vi "Update Status Table by Reference.vi"(8 "error in (no error)":errorcluster, 10 "Plugin Info Array":T1[](array[typedef]) {"Node Status"."Monitor Doubles"."4" format="%#_9g"; "Node Status"."Monitor Doubles"."3" format="%#_9g"; "Node Status"."Monitor Doubles"."2" format="%#_9g"; "Node Status"."Monitor Doubles"."1" format="%#_9g"; "Node Status"."Timing Statistics (us)"."Period"."Avg" format="%_6g"}, 11 "Table Control in":refnum<vi>) -> (0 "error out":errorcluster)   [LabVIEW 2021, in "CIF_UI.lvclass"]
uses:
  CIF_UI.lvclass
  CIFCore/Common/Typedef/PluginInfo.ctl
  CIFCore/Common/Typedef/Version Simple.ctl
  CIFCore/Common/Typedef/gRPC Reported Plugin Status.ctl
  CIFCore/Common/Typedef/Plugin State.ctl
  CIFCore/Common/Typedef/Timing Statistics.ctl
  CIFCore/Common/Typedef/Timing Stats Base.ctl
  CIFCore/Common/Typedef/FIFO Statistics.ctl
  CIFCore/Common/Typedef/Simple Error.ctl
  CIFCore/Common/Typedef/Monitor Doubles.ctl
  CIFCore/Common/Typedef/Monitor U64.ctl
  CIFCore/Common/Typedef/Monitor I64.ctl
  CIFCore/Common/CIFCoreCommon.lvlib
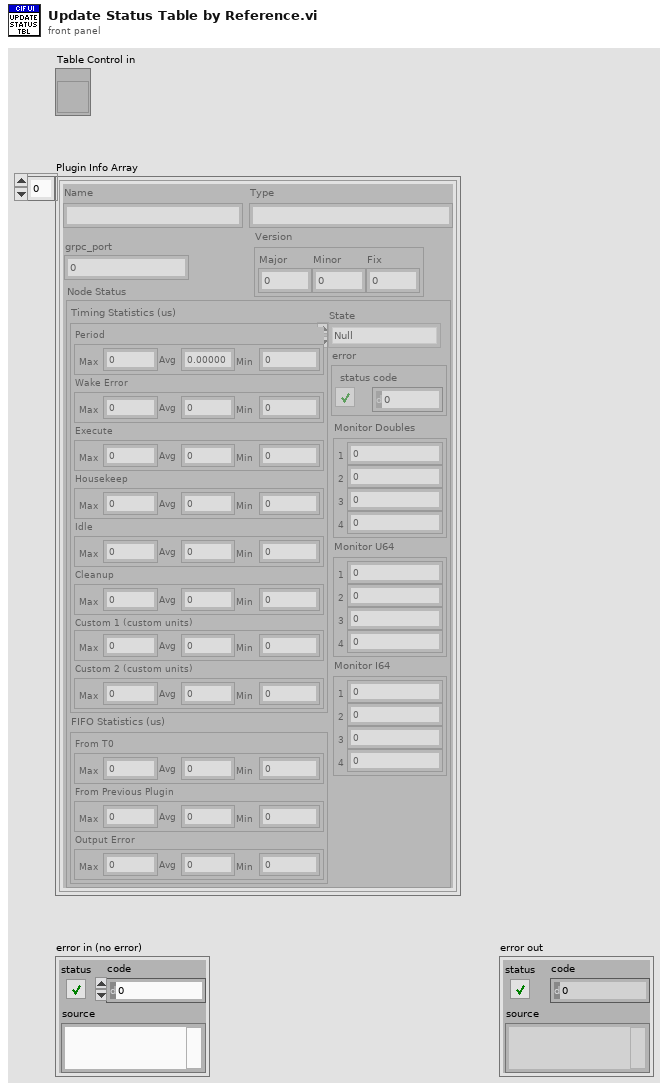
[diagram p1: front panel]
types:
  T1 = typedef "CIFCoreCommon.lvlib/PluginInfo.ctl" = cluster{"Name":string, "Type":string, "grpc_port":i32, "Version":T2, "Node Status":T3}
  T2 = typedef "CIFCoreCommon.lvlib/Version Simple.ctl" = cluster{"Major":i32, "Minor":i32, "Fix":i32}
  T3 = typedef "CIFCoreCommon.lvlib/gRPC Reported Plugin Status.ctl" = cluster{"State":T4, "Timing Statistics (us)":T5, "FIFO Statistics (us)":T7, "error":T8, "Monitor Doubles":T9, "Monitor U64":T10, "Monitor I64":T11}
  T4 = typedef "CIFCoreCommon.lvlib/Plugin State.ctl" = enum32{"Null", "Creating", "Listening", "Running", "CleaningUp", "Destroying"}
  T5 = typedef "CIFCoreCommon.lvlib/Timing Statistics.ctl" = cluster{"Period":T6, "Wake Error":T6, "Execute":T6, "Housekeep":T6, "Idle":T6, "Cleanup":T6, "Custom 1 (custom units)":T6, "Custom 2 (custom units)":T6}
  T6 = typedef "CIFCoreCommon.lvlib/Timing Stats Base.ctl" = cluster{"Max":i64, "Avg":dbl, "Min":i64}
  T7 = typedef "CIFCoreCommon.lvlib/FIFO Statistics.ctl" = cluster{"From T0":T6, "From Previous Plugin":T6, "Output Error":T6}
  T8 = typedef "CIFCoreCommon.lvlib/Simple Error.ctl" = cluster{"status":bool, "code":i32}
  T9 = typedef "CIFCoreCommon.lvlib/Monitor Doubles.ctl" = cluster{"1":dbl, "2":dbl, "3":dbl, "4":dbl}
  T10 = typedef "CIFCoreCommon.lvlib/Monitor U64.ctl" = cluster{"1":u64, "2":u64, "3":u64, "4":u64}
  T11 = typedef "CIFCoreCommon.lvlib/Monitor I64.ctl" = cluster{"1":i64, "2":i64, "3":i64, "4":i64}
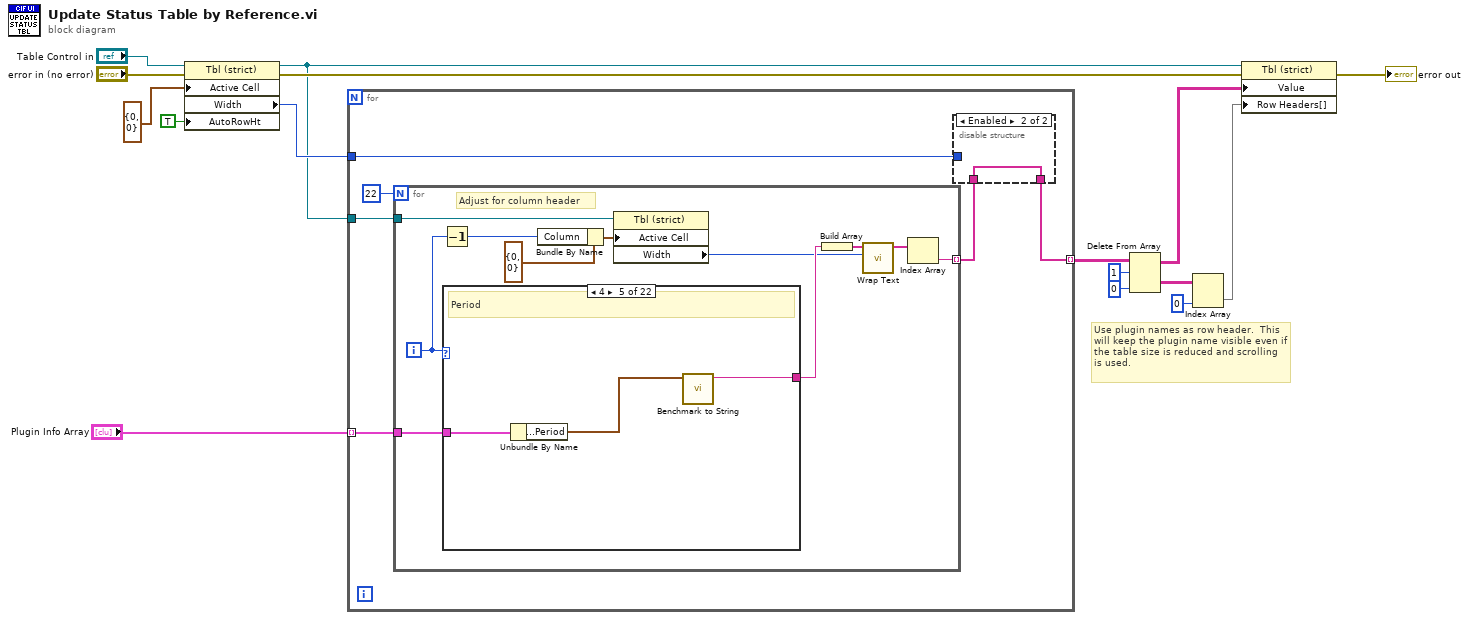
[diagram p0: block diagram]
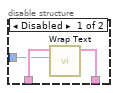
[diagram p2: hidden frame]
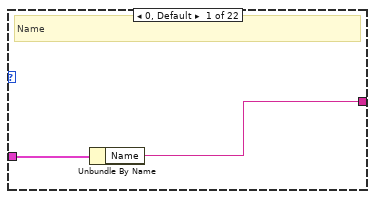
[diagram p3: hidden frame]
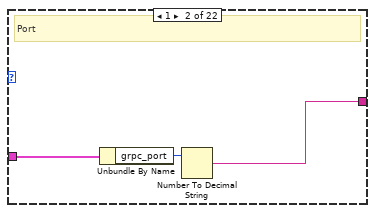
[diagram p4: hidden frame]
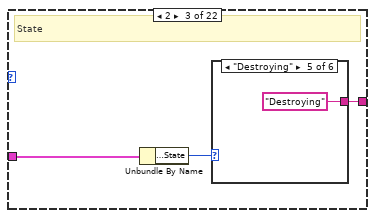
[diagram p5: hidden frame]
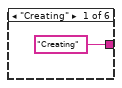
[diagram p6: hidden frame]
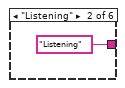
[diagram p7: hidden frame]
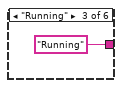
[diagram p8: hidden frame]
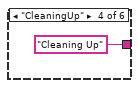
[diagram p9: hidden frame]
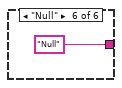
[diagram p10: hidden frame]
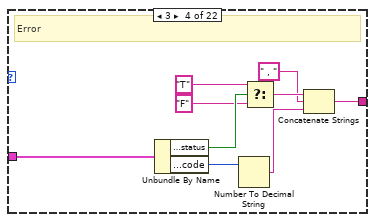
[diagram p11: hidden frame]
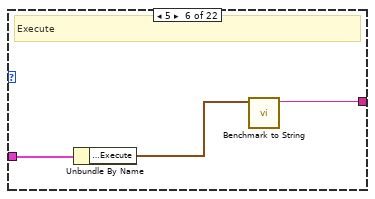
[diagram p12: hidden frame]
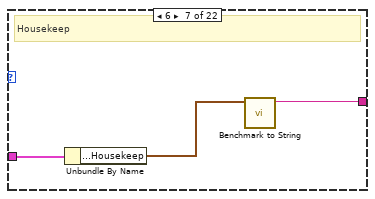
[diagram p13: hidden frame]
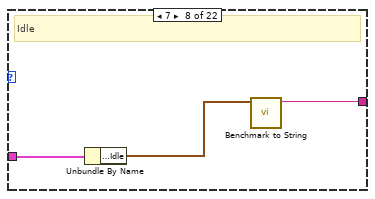
[diagram p14: hidden frame]
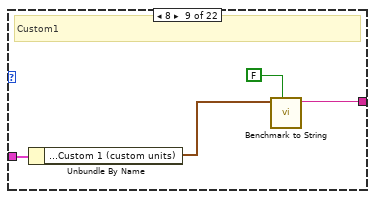
[diagram p15: hidden frame]
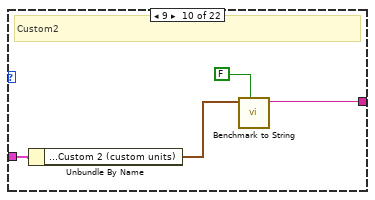
[diagram p16: hidden frame]
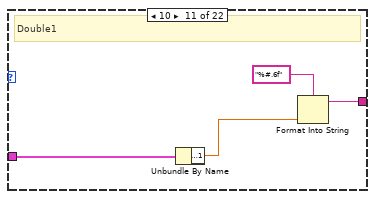
[diagram p17: hidden frame]
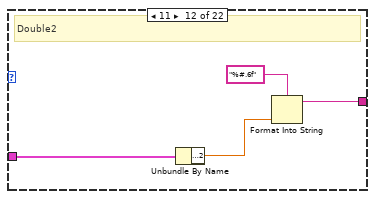
[diagram p18: hidden frame]
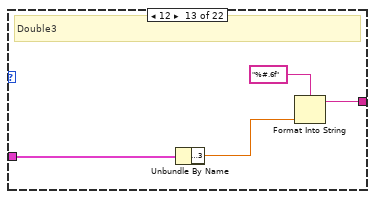
[diagram p19: hidden frame]
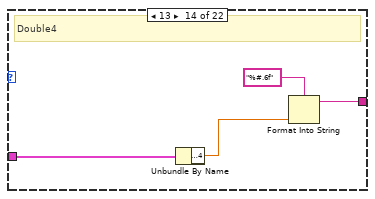
[diagram p20: hidden frame]
diagram:
  # "Use plugin names as row header.  This will keep the plugin name visible even if the table size is reduced and scrolling is used."
  n1 = property on="Property Node" class="Tbl (strict)"(reference="Table Control in", error in="error in (no error)", "Active Cell"=cluster{"Row":i32, "Column":i32} {"Row"=0, "Column"=0}, "AutoRowHt"=TRUE ("Autosizing Row Height")) -> (reference out=w10:refnum<vi>, error out=w13:errorcluster, "Width"=w11:u32)
  n2 = for {
    tunnel: [w19] -> w8 mode=indexing
    tunnel: "Plugin Info Array" -> [w21] mode=indexing
    tunnel: w11 -> [w18]
    tunnel: w10 -> [w17]
    n3 = for {
      N: 22 -> [_]
      tunnel: [w33] -> w20 mode=indexing
      tunnel: w21 -> [w37]
      tunnel: w17 -> [w32]
      i -> [w30]
      # "Adjust for column header"
      n4 = Decrement(x=w30) -> (x-1=w27:i32)
      n5 = case shown="4" w30 {
        tunnel: [w38 w42 w43 w52 w62 w65 w68 w71 w75 w78 w81 w86 w90 w94 w97 w100 w103 w106 w109 w112 w115 w118] -> w34
        tunnel: w37 -> [w39 w41 w45 w60 w63 w66 w69 w72 w76 w80 w84 w88 w92 w96 w99 w102 w105 w108 w111 w114 w117 w120]
        frame 0, Default {
          # "Name"
          n6 = Unbundle By Name(w39) -> ("Name"=w38:string)
        }
        frame 1 {
          # "Port"
          n7 = Unbundle By Name(w41) -> ("grpc_port"=w40:i32)
          n8 = Number To Decimal String(number=w40) -> (decimal integer string=w42:string)  [unwired: 1 in]
        }
        frame 2 {
          # "State"
          n9 = Unbundle By Name(w45) -> ("Node Status.State"=w44:T4)
          n10 = case shown="\"Destroying\"" w44 {
            tunnel: ["Creating" "Listening" "Running" "Cleaning Up" "Destroying" "Null"] -> w43
            frame "Creating" {
            }
            frame "Listening" {
            }
            frame "Running" {
            }
            frame "CleaningUp" {
            }
            frame "Destroying" {
            }
            frame "Null" {
            }
          }
        }
        frame 3 {
          # "Error"
          n11 = Unbundle By Name(w60) -> ("Node Status.error.status"=w58:bool, "Node Status.error.code"=w59:i32)
          n12 = Number To Decimal String(number=w59) -> (decimal integer string=w53:string)  [unwired: 1 in]
          n13 = Select(t="T", s=w58, f="F") -> (s? t:f=w55:string)
          n14 = Concatenate Strings(w55, " , ", w53) -> (w52:string)
        }
        frame 4 {
          # "Period"
          n15 = Unbundle By Name(w63) -> ("Node Status.Timing Statistics (us).Period"=w61:T6)
          n16 = call "Benchmark to String.vi"("Timing Stats"=w61) -> ("concatenated string"=w62:string)  [unwired: 10 in]
        }
        frame 5 {
          # "Execute"
          n17 = Unbundle By Name(w66) -> ("Node Status.Timing Statistics (us).Execute"=w64:T6)
          n18 = call "Benchmark to String.vi"("Timing Stats"=w64) -> ("concatenated string"=w65:string)  [unwired: 10 in]
        }
        frame 6 {
          # "Housekeep"
          n19 = Unbundle By Name(w69) -> ("Node Status.Timing Statistics (us).Housekeep"=w67:T6)
          n20 = call "Benchmark to String.vi"("Timing Stats"=w67) -> ("concatenated string"=w68:string)  [unwired: 10 in]
        }
        frame 7 {
          # "Idle"
          n21 = Unbundle By Name(w72) -> ("Node Status.Timing Statistics (us).Idle"=w70:T6)
          n22 = call "Benchmark to String.vi"("Timing Stats"=w70) -> ("concatenated string"=w71:string)  [unwired: 10 in]
        }
        frame 8 {
          # "Custom1"
          n23 = Unbundle By Name(w76) -> ("Node Status.Timing Statistics (us).Custom 1 (custom units)"=w74:T6)
          n24 = call "Benchmark to String.vi"("Divide/1k"=FALSE, "Timing Stats"=w74) -> ("concatenated string"=w75:string)  [unwired: 9 in]
        }
        frame 9 {
          # "Custom2"
          n25 = Unbundle By Name(w80) -> ("Node Status.Timing Statistics (us).Custom 2 (custom units)"=w79:T6)
          n26 = call "Benchmark to String.vi"("Divide/1k"=FALSE, "Timing Stats"=w79) -> ("concatenated string"=w78:string)  [unwired: 9 in]
        }
        frame 10 {
          # "Double1"
          n27 = Unbundle By Name(w84) -> ("Node Status.Monitor Doubles.1"=w82:dbl)
          n28 = Format Into String(format string="%#.6f", w82) -> (resulting string=w81:string)  [unwired: 2 in, 1 out]
        }
        frame 11 {
          # "Double2"
          n29 = Unbundle By Name(w88) -> ("Node Status.Monitor Doubles.2"=w85:dbl)
          n30 = Format Into String(format string="%#.6f", w85) -> (resulting string=w86:string)  [unwired: 2 in, 1 out]
        }
        frame 12 {
          # "Double3"
          n31 = Unbundle By Name(w92) -> ("Node Status.Monitor Doubles.3"=w89:dbl)
          n32 = Format Into String(format string="%#.6f", w89) -> (resulting string=w90:string)  [unwired: 2 in, 1 out]
        }
        frame 13 {
          # "Double4"
          n33 = Unbundle By Name(w96) -> ("Node Status.Monitor Doubles.4"=w93:dbl)
          n34 = Format Into String(format string="%#.6f", w93) -> (resulting string=w94:string)  [unwired: 2 in, 1 out]
        }
        frame 14 {
          # "U64_1"
          n35 = Unbundle By Name(w99) -> ("Node Status.Monitor U64.1"=w98:u64)
          n36 = Number To Decimal String(number=w98) -> (decimal integer string=w97:string)  [unwired: 1 in]
        }
        frame 15 {
          # "U64_2"
          n37 = Unbundle By Name(w102) -> ("Node Status.Monitor U64.2"=w101:u64)
          n38 = Number To Decimal String(number=w101) -> (decimal integer string=w100:string)  [unwired: 1 in]
        }
        frame 16 {
          # "U64_3"
          n39 = Unbundle By Name(w105) -> ("Node Status.Monitor U64.3"=w104:u64)
          n40 = Number To Decimal String(number=w104) -> (decimal integer string=w103:string)  [unwired: 1 in]
        }
        frame 17 {
          # "U64_4"
          n41 = Unbundle By Name(w108) -> ("Node Status.Monitor U64.4"=w107:u64)
          n42 = Number To Decimal String(number=w107) -> (decimal integer string=w106:string)  [unwired: 1 in]
        }
        frame 18 {
          # "I64_1"
          n43 = Unbundle By Name(w111) -> ("Node Status.Monitor I64.1"=w110:i64)
          n44 = Number To Decimal String(number=w110) -> (decimal integer string=w109:string)  [unwired: 1 in]
        }
        frame 19 {
          # "I64_2"
          n45 = Unbundle By Name(w114) -> ("Node Status.Monitor I64.2"=w113:i64)
          n46 = Number To Decimal String(number=w113) -> (decimal integer string=w112:string)  [unwired: 1 in]
        }
        frame 20 {
          # "I64_3"
          n47 = Unbundle By Name(w117) -> ("Node Status.Monitor I64.3"=w116:i64)
          n48 = Number To Decimal String(number=w116) -> (decimal integer string=w115:string)  [unwired: 1 in]
        }
        frame 21 {
          # "I64_4"
          n49 = Unbundle By Name(w120) -> ("Node Status.Monitor I64.4"=w119:i64)
          n50 = Number To Decimal String(number=w119) -> (decimal integer string=w118:string)  [unwired: 1 in]
        }
      }
      n51 = Bundle By Name(cluster=cluster{"Row":i32, "Column":i32} {"Row"=0, "Column"=0} ("Active Cell"), "Column"=w27) -> (w28:cluster{"Row":i32, "Column":i32})
      n52 = property on="Property Node" class="Tbl (strict)"(reference=w32, "Active Cell"=w28) -> ("Width"=w29:u32)  [unwired: 1 in, 2 out]
      n53 = Build Array(w34) -> (w36:string[])
      n54 = call "Wrap Text.vi"("width"=w29, "item names"=w36) -> ("item names with wrapping"=w35:string[])  [unwired: 8 in, 1 out]
      n55 = Index Array(array=w35) -> (element=w33:string)  [unwired: 1 in]
    }
    n56 = disable-structure shown="Enabled" {
      disable-tunnel: w20 -> [w25 w26]
      disable-tunnel: [w24 w26] -> w19
      disable-tunnel: w18 -> [w23 _]
      frame Disabled {
        n57 = call "Wrap Text.vi"("width"=w23, "item names"=w25) -> ("item names with wrapping"=w24:string[])  [unwired: 8 in, 1 out]
      }
      frame Enabled {
      }
    }
  }
  n58 = Delete From Array(array=w8, length=1, index (col)=0 ("disabled index (col)")) -> (deleted portion=w5:string[][], array with subset deleted=w6:string[][])  [unwired: 1 in]
  n59 = Index Array(array=w5, index (col)=0 ("disabled index (col)")) -> (element=w4:string[])  [unwired: 1 in]
  n60 = property class="Tbl (strict)"(reference=w10, error in=w13, "Value"=w6, "Row Headers[]"=w4) -> (error out=→"error out":errorcluster)  [unwired: 1 out]
